vi "Housekeeping.vi"(8 "error in (no error)":errorcluster, 11 "CIFTemplatePlugin in":refnum<class "CIFTemplatePlugin.lvclass">) -> (0 "error out":errorcluster, 3 "CIFTemplatePlugin out":refnum<class "CIFTemplatePlugin.lvclass">)   [LabVIEW 2021, in "CIFTemplatePlugin.lvclass"]
uses:
  CIFTemplatePlugin.lvclass
  CIFTemplatePlugin.lvclass/CIFTemplatePlugin.ctl
  CIFCore/Class/CIFCorePlugin.lvclass
  CIFCore/Class/Typedef/Energized States.ctl
  D:/dev/CIF-LVCore/src/CIFCore/Class/CIFCorePlugin.lvclass
  D:/dev/CIF-LVCore/src/CIFTemplatePlugin/Class/CIFTemplatePlugin.lvclass
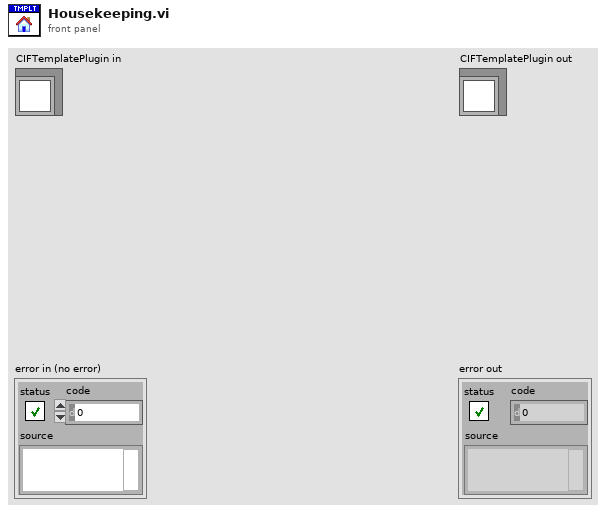
[diagram p1: front panel]
types:
  T1 = typedef "CIFCorePlugin.lvclass/Energized States.ctl" = enum16{"Listen", "Prepare", "Execute", "Housekeep", "Cleanup", "Destroy"}
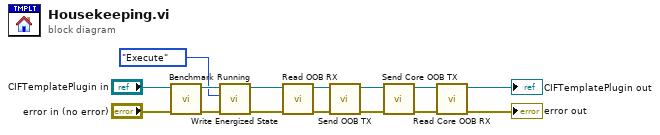
[diagram p0: block diagram]
diagram:
  n1 = call "Benchmark Running.vi"("error in (no error)"="error in (no error)", "CIFCorePlugin in"="CIFTemplatePlugin in") -> ("error out"=w13:errorcluster, "CIFCorePlugin out"=w12:refnum<class "CIFTemplatePlugin.lvclass">)  [unwired: 8 in]
  n2 = call "Write Energized State.vi"("error in (no error)"=w13, "Energized State"=Energized_States."Execute", "CIFCorePlugin in"=w12) -> ("error out"=w8:errorcluster, "CIFCorePlugin out"=w9:refnum<class "CIFTemplatePlugin.lvclass">)  [unwired: 7 in]
  n3 = call "Read OOB RX.vi"("error in (no error)"=w8, "CIFTemplatePlugin in"=w9) -> ("error out"=w10:errorcluster, "CIFTemplatePlugin out"=w7:refnum<class "CIFTemplatePlugin.lvclass">)  [unwired: 8 in]
  n4 = call "Send OOB TX.vi"("error in (no error)"=w10, "CIFTemplatePlugin in"=w7) -> ("error out"=w5:errorcluster, "CIFTemplatePlugin out"=w6:refnum<class "CIFTemplatePlugin.lvclass">)  [unwired: 8 in]
  n5 = call "Send Core OOB TX.vi"("error in (no error)"=w5, "CIFCorePlugin in"=w6) -> ("error out"=w14:errorcluster, "CIFCorePlugin out"=w15:refnum<class "CIFTemplatePlugin.lvclass">)  [unwired: 8 in]
  n6 = call "Read Core OOB RX.vi"("error in (no error)"=w14, "CIFCorePlugin in"=w15) -> ("error out"=→"error out":errorcluster, "CIFCorePlugin out"=→"CIFTemplatePlugin out":refnum<class "CIFTemplatePlugin.lvclass">)  [unwired: 8 in]
